vi "FPGA_Fgen.vi"() -> ()   [LabVIEW 2018]
uses:
  <vilib>/Platform/TimedLoop/XDataNode/timing_clust.ctl
  <vilib>/Platform/TimedLoop/XDataNode/nitl_modes.ctl
  <vilib>/Platform/TimedLoop/XDataNode/wakeup.ctl
  <vilib>/rvi/Emulation/niFpgaSctlEmulationGetInTimedLoop.vi
  <vilib>/rvi/Emulation/niFpgaEmulationReportErrorSimple.vi
  <vilib>/rvi/Emulation/niFpgaGetClockAttributes.vi
  <vilib>/rvi/Emulation/niFpgaCriticalErrorInLSC.vi
  <vilib>/rvi/Memory/Memory_Emulation/nirvimemoryFastEmulation.vi
  <vilib>/rvi/Memory/Memory_Emulation/nirvimemoryEmulation.vi
  <vilib>/rvi/Emulation/niFpgaEmulationIsFPGAContextNoSignature.vi
  <vilib>/rvi/DataTransferAndStorage/Container/Common/niFpgaContainerGetUniqueNameForEmu.vi
  <vilib>/rvi/Emulation/niFpgaProcessEmulError.vi
  <vilib>/rvi/errors/nirviReportUnexpectedCaseInternalError (U32).vi
  <vilib>/rvi/errors/niFpgaSetErrorForExecOnDevCompSimple.vi
  <vilib>/rvi/eio/common/nirviEmuReportErrorAndStop.vi
  <vilib>/rvi/FIFO/Fifo_Resource/nirvififoEmulationSetSize.vi
  <vilib>/rvi/FIFO/Fifo_Resource/nirviFifoEmulationQueueMgr.vi
  <instcachedir>/0/nirviFifoEmulationQueueMgr_E5CAEC123FF24DC58D834DCA3CDAA9B5.lvgen/nirviFifoEmulationQueueMgr_E5CAEC123FF24DC58D834DCA3CDAA9B5_003.vi
  <vilib>/rvi/FIFO/Fifo_Resource/nirvififoEmulationDetermineInputValidOut.vi
  <vilib>/rvi/FIFO/Fifo_Resource/nirvififoEmulationCreateLock.vi
  <vilib>/rvi/FIFO/Fifo_Resource/nirvififoEmulationObtainLock.vi
  <vilib>/rvi/FIFO/Fifo_Resource/nirvififoEmulationReleaseLock.vi
  <vilib>/rvi/occurrence/nirviWaitOnOccurrenceBase.vi
  <vilib>/rvi/errors/nirviReportUnexpectedCaseInternalError.vi
  <vilib>/Utility/error.llb/Clear Errors.vi
  <vilib>/Platform/TimedLoop/XDataNode/XDataNode.xnode
  <vilib>/rvi/DataTransferAndStorage/Container/XNode/niFpgaContainer.xnode
  <vilib>/rvi/FIFO/Fifo_Resource/nirvififoEmulationWrite.vi
  <vilib>/rvi/FIFO/Fifo_Resource/nirvififoEmulationRead.vi
  <vilib>/Platform/TimedLoop/XDataNode/XDNodeRunTimeDep.lvlib
panel:
  in  "DeCyc":u32
  in  "Amp":u16
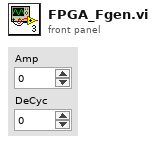
[diagram p1: front panel]
types:
  T1 = typedef "XDNodeRunTimeDep.lvlib/timing_clust.ctl" = cluster{"Expected End [f-1]":u64, "Actual End [f-1]":u64, "Finished Late? [f-1]":bool, "Expected End [i-1]":u64, "Actual End [i-1]":u64, "Finished Late? [i-1]":bool, "Expected Start [i]":u64, "Actual Start [i]":u64, "Expected Start [f]":u64, "Actual Start [f]":u64, "Source Name":string, "Structure Name":string, "Period":i64, "Deadline":i64, "Offset":i64, "Start":i64, "Priority":i32, "Timeout":i32, "Mode":T2, "Wakeup Reason":T3, "Error":errorcluster, "Source Type":string, "Secondary Source Type":string, "Global End Time":u64, "Global Start Time":u64, "Frame Duration":u64, "Iteration Duration":u64, "Assigned CPU":i32, "I/O Scan Engine Mode":u32}
  T2 = typedef "XDNodeRunTimeDep.lvlib/nitl_modes.ctl" = enum32{"No Change", "Process missed periods, maintain original phase", "Discard missed periods, maintain original phase", "Process missed periods, ignore original phase", "Discard missed periods, ignore original phase"}
  T3 = typedef "XDNodeRunTimeDep.lvlib/wakeup.ctl" = enum32{"Normal", "Aborted", "Asynchronous wakeup", "Timing source error", "Timed loop error", "Timeout"}
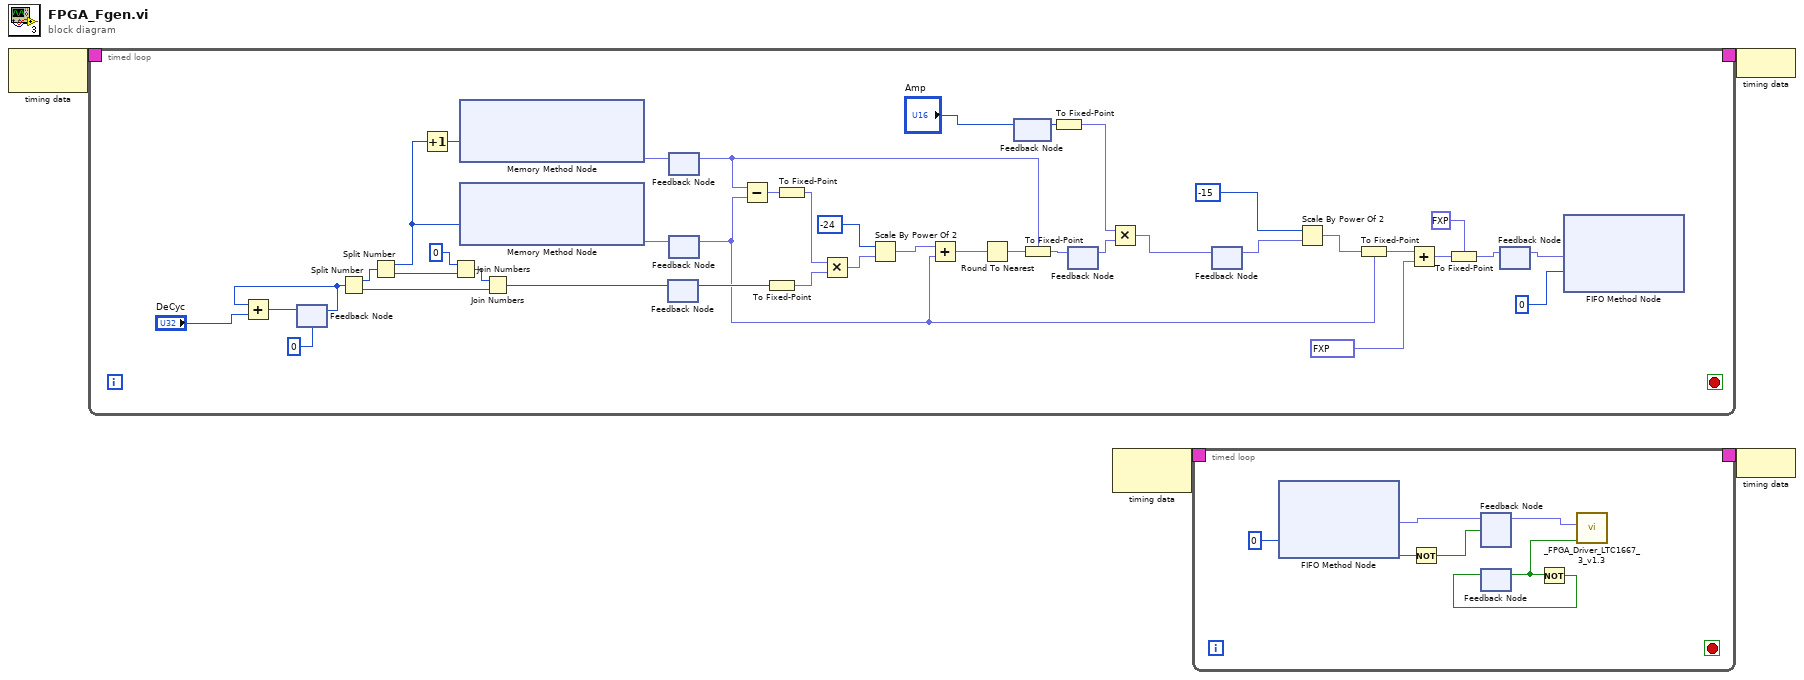
[diagram p0: block diagram]
diagram:
  n1 = node-c288() -> (w4:T1)  [unwired: 1 in]
  n2 = timed-loop {
    timing: w4 -> [_]
    timing-out: [_] -> w3
    stop <- _ stop-if-true
    n3 = feedback #1(u32 0) -> (w39:u32)
    n4 = Add(x=w39, y="DeCyc") -> (x+y=w40:u32)
    n5 = feedback-in #1(w40) -> ()
    n6 = Split Number(x=w39) -> (hi(x)=w44:u16, lo(x)=w34:u16)
    n7 = Split Number(x=w44) -> (hi(x)=w38:u8, lo(x)=w37:u8)
    n8 = Increment(x=w38) -> (x+1=w43:u8)
    n9 = Join Numbers(hi=u8 0, lo=w37) -> ((hi.lo)=w35:u16)
    n10 = xnode ("Memory Method Node")("Address A"=w43) -> ("Data A"=w42:fxp<+/-,28,14>)  [unwired: 1 in, 1 out]
    n11 = xnode ("Memory Method Node")("Address B"=w38) -> ("Data B"=w41:fxp<+/-,28,14>)  [unwired: 1 in, 1 out]
    n12 = Join Numbers(hi=w35, lo=w34) -> ((hi.lo)=w33:u32)
    n13 = feedback-in #2(w33) -> ()
    n14 = feedback #2() -> (w24:u32)  [unwired: 1 in]
    n15 = feedback-in #3(w42) -> ()
    n16 = feedback #3() -> (w21:fxp<+/-,28,14>)  [unwired: 1 in]
    n17 = feedback-in #4(w41) -> ()
    n18 = feedback #4() -> (w13:fxp<+/-,28,14>)  [unwired: 1 in]
    n19 = Subtract(x=w21, y=w13) -> (x-y=w23:fxp<+/-,29,15>)
    n20 = To Fixed-Point(number=w24) -> (fixed-point=w32:fxp<+,24,24>)  [unwired: 1 in]
    n21 = To Fixed-Point(number=w23) -> (fixed-point=w22:fxp<+/-,23,9>)  [unwired: 1 in]
    n22 = Multiply(x=w22, y=w32) -> (x*y=w31:fxp<+/-,47,33>)
    n23 = Scale By Power Of 2(n=i16 -24, x=w31) -> (x*2^n=w29:fxp<+/-,47,33>)
    n24 = Add(x=w29, y=w13) -> (x+y=w25:fxp<+/-,48,34>)
    n25 = Round To Nearest(number=w25) -> (nearest integer value=w28:fxp<+/-,34,34>)
    n26 = feedback-in #5("Amp") -> ()
    n27 = feedback #5() -> (w19:u16)  [unwired: 1 in]
    n28 = To Fixed-Point(fixed-point type=w21, number=w28) -> (fixed-point=w27:fxp<+/-,28,14>)
    n29 = To Fixed-Point(number=w19) -> (fixed-point=w18:fxp<+,32,32>)  [unwired: 1 in]
    n30 = feedback-in #6(w27) -> ()
    n31 = feedback #6() -> (w20:fxp<+/-,28,14>)  [unwired: 1 in]
    n32 = Multiply(x=w18, y=w20) -> (x*y=w17:fxp<+/-,60,46>)
    n33 = feedback-in #7(w17) -> ()
    n34 = feedback #7() -> (w16:fxp<+/-,60,46>)  [unwired: 1 in]
    n35 = Scale By Power Of 2(n=i16 -15, x=w16) -> (x*2^n=w14:fxp<+/-,60,46>)
    n36 = To Fixed-Point(fixed-point type=w13, number=w14) -> (fixed-point=w12:fxp<+/-,28,14>)
    n37 = Add(x=w12, y=fxp<+/-,28,14> 8191.5) -> (x+y=w10:fxp<+/-,29,15>)
    n38 = To Fixed-Point(fixed-point type=fxp<+,14,14> 0.0 ("Element"), number=w10) -> (fixed-point=w8:fxp<+,14,14>)
    n39 = feedback #8() -> (w7:fxp<+,14,14>)  [unwired: 1 in]
    n40 = feedback-in #8(w8) -> ()
    n41 = xnode ("FIFO Method Node")("Element"=w7, "Timeout"=0) -> ()  [unwired: 1 in, 2 out]
  }
  n42 = node-c288() -> (w2:T1)  [unwired: 1 in]
  n43 = timed-loop {
    timing: w2 -> [_]
    timing-out: [_] -> w1
    stop <- _ stop-if-true
    n44 = xnode ("FIFO Method Node")("Timeout"=0) -> ("Element"=w50:fxp<+/-,16,14>, "Timed Out?"=w52:bool)  [unwired: 1 in, 1 out]
    n45 = Not(x=w52) -> (.not. x?=w51:bool)
    n46 = feedback-in #9(w50, w51) -> ()
    n47 = feedback #9() -> (w49:fxp<+/-,16,14>)  [unwired: 1 in]
    n48 = feedback #10() -> (w53:bool)  [unwired: 1 in]
    n49 = Not(x=w53) -> (.not. x?=w54:bool)
    n50 = feedback-in #10(w54) -> ()
    n51 = call "_FPGA_Driver_LTC1667_3_v1.3.vi"("Clk"=w53, "Data_in"=w49) -> ()  [unwired: 10 in]
  }
  n52 = node-c288(w3) -> ()
  n53 = node-c288(w1) -> ()
